vi "main local variable.vi"() -> ()   [LabVIEW 2019]
uses:
  Controls/semafor.ctl
  Controls/Estats.ctl
panel:
  out "Semafor":T1
  out "pedestrian":bool
  in  "SET":bool
  in  "stop":bool
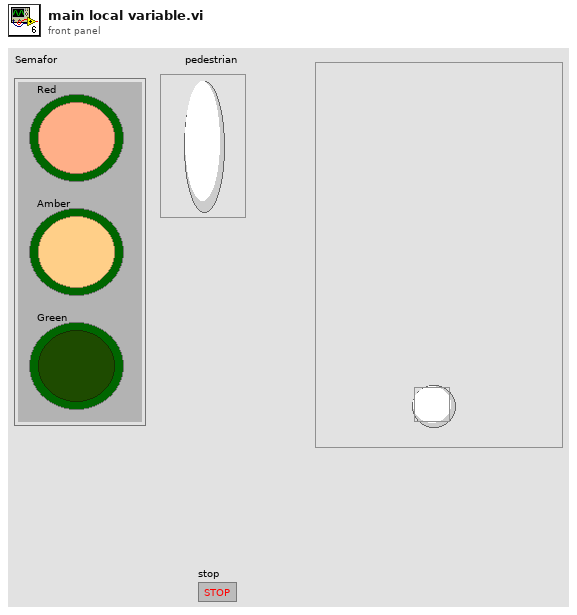
[diagram p1: front panel]
types:
  T1 = typedef "semafor.ctl" = cluster{"Red":bool, "Amber":bool, "Green":bool}
  T2 = typedef "Estats.ctl" = enum16{"Init", "Green", "Amber-red", "red", "amber"}
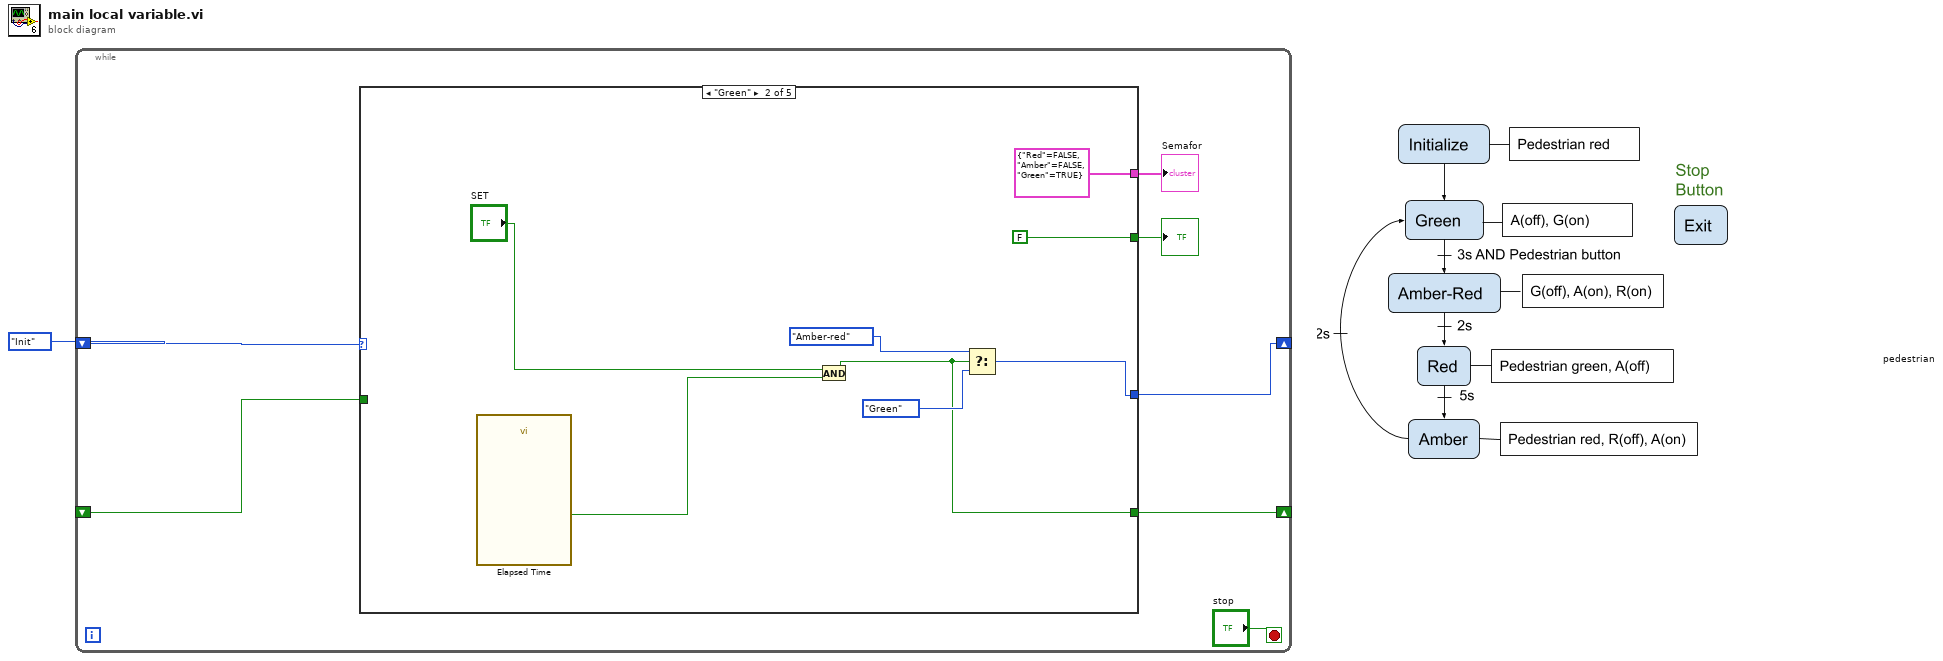
[diagram p0: block diagram]
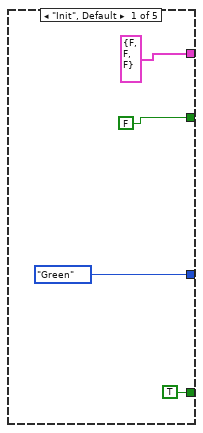
[diagram p2: hidden frame]
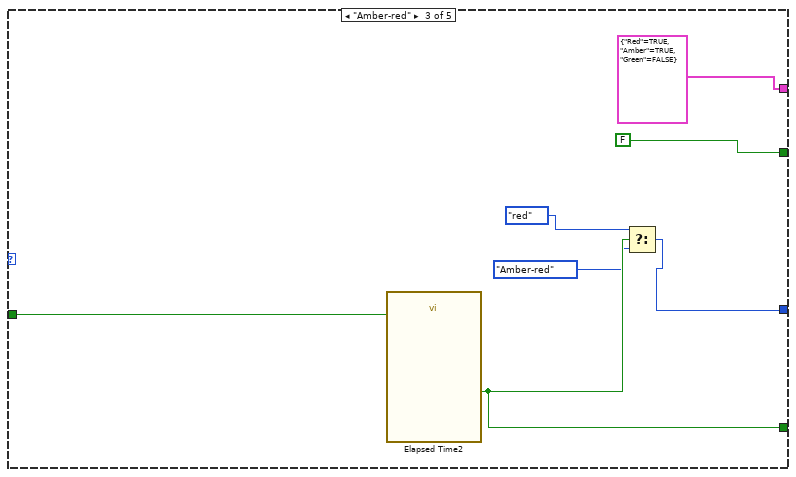
[diagram p3: hidden frame]
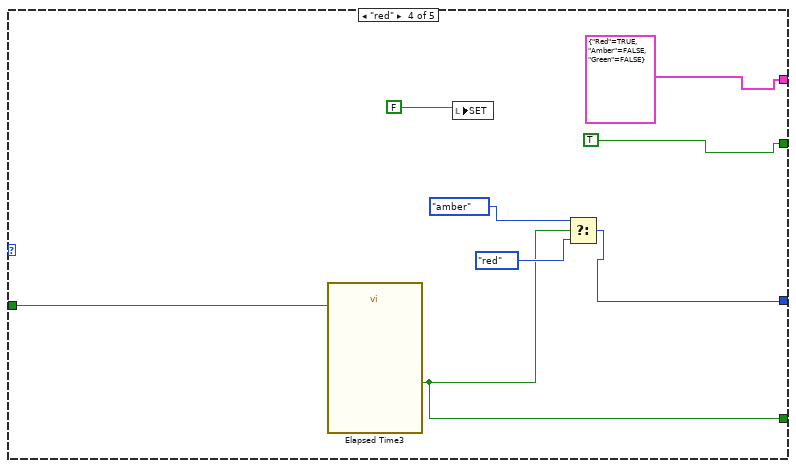
[diagram p4: hidden frame]
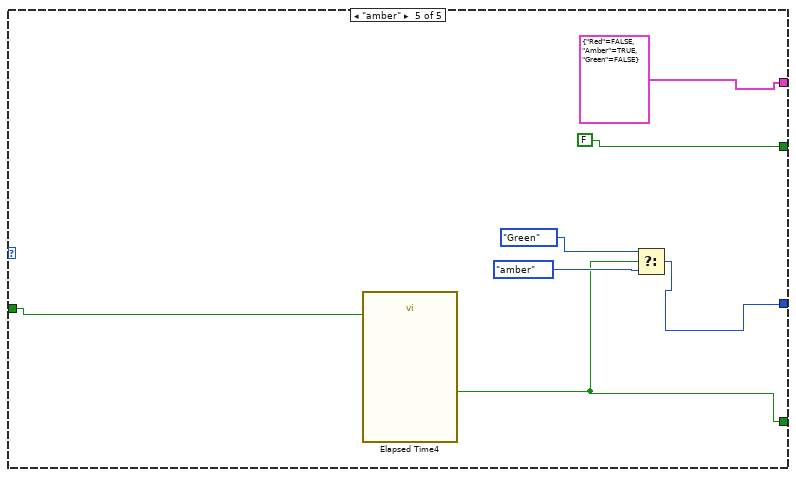
[diagram p5: hidden frame]
diagram:
  n1 = while {
    shift-right: [w7] -> _
    shift-left: _ -> [w6]
    shift-right: [w3] -> _
    shift-left: Estats."Init" ("Enum") -> [w4]
    stop <- "stop" stop-if-true
    n2 = case shown="\"Green\"" w4 {
      tunnel: [Estats."Green" ("Enum") w17 w27 w33 w40] -> w3
      tunnel: [TRUE ("Time has Elapsed") w13 w25 w32 w39] -> w7
      tunnel: w6 -> [_ _ w23 w31 w38]
      tunnel: [T1 {"Red"=FALSE, "Amber"=FALSE, "Green"=FALSE} ("Semafor") T1 {"Red"=FALSE, "Amber"=FALSE, "Green"=TRUE} ("Semafor") T1 {"Red"=TRUE, "Amber"=TRUE, "Green"=FALSE} ("Semafor") T1 {"Red"=TRUE, "Amber"=FALSE, "Green"=FALSE} ("Semafor") T1 {"Red"=FALSE, "Amber"=TRUE, "Green"=FALSE} ("Semafor")] -> w5
      tunnel: [FALSE ("pedestrian") FALSE ("pedestrian") FALSE ("pedestrian") TRUE ("pedestrian") FALSE ("pedestrian")] -> w2
      frame "Init", Default {
      }
      frame "Green" {
        n3 = call "Elapsed Time"() -> ("Time has Elapsed"=w18:bool)  [unwired: 12 in, 7 out]
        n4 = And(x="SET", y=w18) -> (x .and. y?=w13:bool)
        n5 = Select(t=Estats."Amber-red" ("Enum"), s=w13, f=Estats."Green" ("Enum")) -> (s? t:f=w17:T2)
      }
      frame "Amber-red" {
        n6 = call "Elapsed Time2"("Reset"=w23) -> ("Time has Elapsed"=w25:bool)  [unwired: 11 in, 7 out]
        n7 = Select(t=Estats."red" ("Enum"), s=w25, f=Estats."Amber-red" ("Enum")) -> (s? t:f=w27:T2)
      }
      frame "red" {
        n8 = call "Elapsed Time3"("Reset"=w31) -> ("Time has Elapsed"=w32:bool)  [unwired: 11 in, 7 out]
        n9 = local write "SET"(FALSE ("pedestrian")) -> ()
        n10 = Select(t=Estats."amber" ("Enum"), s=w32, f=Estats."red" ("Enum")) -> (s? t:f=w33:T2)
      }
      frame "amber" {
        n11 = call "Elapsed Time4"("Reset"=w38) -> ("Time has Elapsed"=w39:bool)  [unwired: 11 in, 7 out]
        n12 = Select(t=Estats."Green" ("Enum"), s=w39, f=Estats."amber" ("Enum")) -> (s? t:f=w40:T2)
      }
    }
    "Semafor" <- w5
    "pedestrian" <- w2
  }
